vi "FullSpeedAndRun 2 SpeedIndicator (uSMC).vi"(4 "run":bool, 5 "full speed":bool) -> (1 "speed":u16)   [LabVIEW 2010, in "SignalWriterMH110203USBStepperMotor.lvclass"]
uses:
  SignalWriterMH110203USBStepperMotor.lvclass
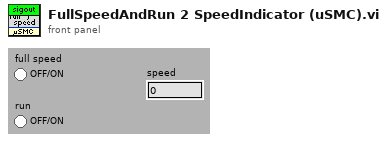
[diagram p1: front panel]
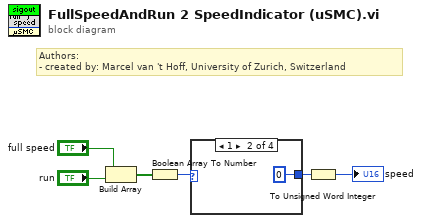
[diagram p0: block diagram]
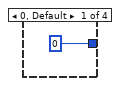
[diagram p2: hidden frame]
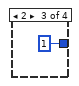
[diagram p3: hidden frame]
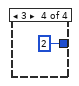
[diagram p4: hidden frame]
diagram:
  # "Authors: \n- created by: Marcel van 't Hoff, University of Zurich, Switzerland"
  n1 = Build Array("full speed", "run") -> (w4:bool[])
  n2 = Boolean Array To Number(Boolean array=w4) -> (number=w3:u32)
  n3 = case shown="1" w3 {
    tunnel: [0 0 1 2] -> w2
    frame 0, Default {
    }
    frame 1 {
    }
    frame 2 {
    }
    frame 3 {
    }
  }
  n4 = To Unsigned Word Integer(number=w2) -> (unsigned 16bit integer=→"speed":u16)
